vi "getGlyphFile.vi"(8 "error in (no error)":errorcluster, 11 "Channel in":refnum<class "Parameter.lvclass">) -> (0 "error out":errorcluster, 2 "Glyph File":string, 3 "Channel out":refnum<class "Parameter.lvclass">)   [LabVIEW 2013, in "Parameter.lvclass"]
doc: "Dynamic Dispatch VI. Returns the name of the glyph file to be used as a glyph in the tree control. A empty string means no glyph."
uses:
  Parameter.lvclass
  Parameter.lvclass/Parameter.ctl
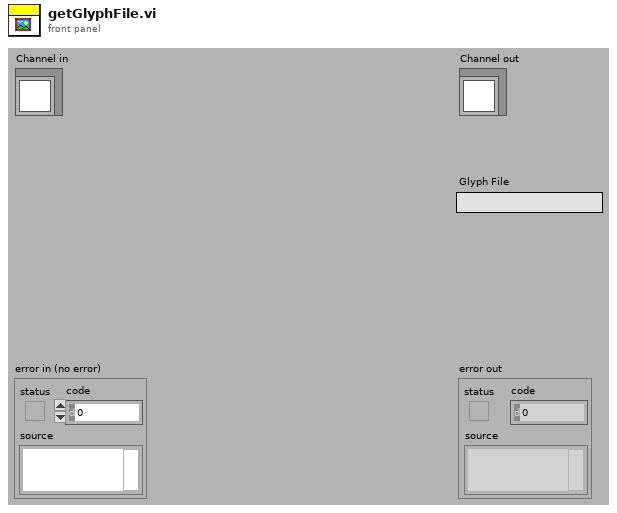
[diagram p1: front panel]
types:
  T1 = typedef "Parameter.lvclass/channel_dataType.ctl" = enum16{"Boolean", "U8", "I8", "U16", "I16", "U32", "I32", "U64", "I64", "FXPI32", "FXPU32", "FXPI64", "FXPU64", "PWM"}
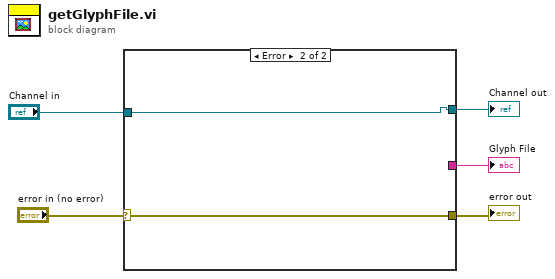
[diagram p0: block diagram]
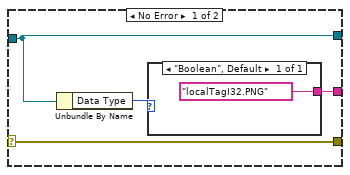
[diagram p2: hidden frame]
diagram:
  n1 = case shown="Error" "error in (no error)" {
    selector: "error in (no error)" -> [w7 w11]
    tunnel: "Channel in" -> [w9 w12]
    tunnel: [w9 w12] -> w3
    tunnel: [w7 w11] -> w2
    tunnel: [w6 _] -> w1
    frame No Error {
      n2 = Unbundle By Name(w9) -> ("Data Type"=w8:T1)
      n3 = case shown="\"Boolean\", Default" w8 {
        tunnel: ["localTagI32.PNG"] -> w6
        frame "Boolean", Default {
        }
      }
    }
    frame Error {
    }
  }
  "error out" <- w2
  "Channel out" <- w3
  "Glyph File" <- w1
